vi "Wrapper.vi"(8 "error in":errorcluster, 10 "Actor in":refnum<class "Actor.lvclass">, 11 "Update Heater DC MSG in":refnum<class "Update Heater DC MSG.lvclass">) -> (0 "error out":errorcluster, 3 "Actor out":refnum<class "Actor.lvclass">)   [LabVIEW 2017, in "Controller.lvlib" / "Update Heater DC MSG.lvclass"]
uses:
  Update Heater DC MSG.lvclass
  <vilib>/ActorFramework/Actor/Actor.lvclass
  Update Heater DC MSG.lvclass/Update Heater DC MSG.ctl
  gController.lvclass
  C:/Program Files (x86)/National Instruments/LabVIEW 2017/vi.lib/MSR Consulting, LLC/General Reuse/SuperActor/SuperActor.lvclass
  C:/Program Files (x86)/National Instruments/LabVIEW 2017/vi.lib/ActorFramework/Actor/Actor.lvclass
  <vilib>/MSR Consulting, LLC/General Reuse/SuperActor/SuperActor.lvclass/SuperActor.ctl
  <vilib>/MSR Consulting, LLC/General Reuse/SuperActor/Read CVT Session.vi
  <vilib>/MSR Consulting, LLC/General Reuse/SuperActor/Read Log Session.vi
  Global DO.vi
  <vilib>/Utility/error.llb/Error Cluster From Error Code.vi
  <vilib>/rvi/errors/niLvFpgaAdjustHostInterfaceError.vi
  <vilib>/MSR Consulting, LLC/General Reuse/Session APIs/_Session Fwk/Session - Root.lvclass
  <vilib>/rvi/interface/nirviReadWriteControl/nirviReadWriteControl.xnode
  FPGA Ref.ctl
  FPGA Bitfiles/server.lvbitx
  <vilib>/MSR Consulting, LLC/General Reuse/Session APIs/CVT/CVT.lvclass
  <vilib>/MSR Consulting, LLC/General Reuse/Session APIs/Session Log/System Log.lvclass
  NiFpgaLv.dll
panel:
  out "x-y 3":u32
  out "x-y 2":u32
  out "x+1":i32
  out "x-y":u32
  out "32-bit output":u32
  out "crd":u8
  out "pas2":u8
  out "pas1":u8
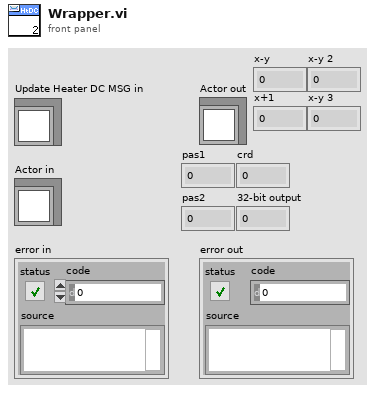
[diagram p1: front panel]
types:
  T1 = typedef "Session - Root.lvclass/Session Handle.ctl" = refnum<data-value>
  T2 = typedef "FPGA Ref.ctl" = refnum<k20>
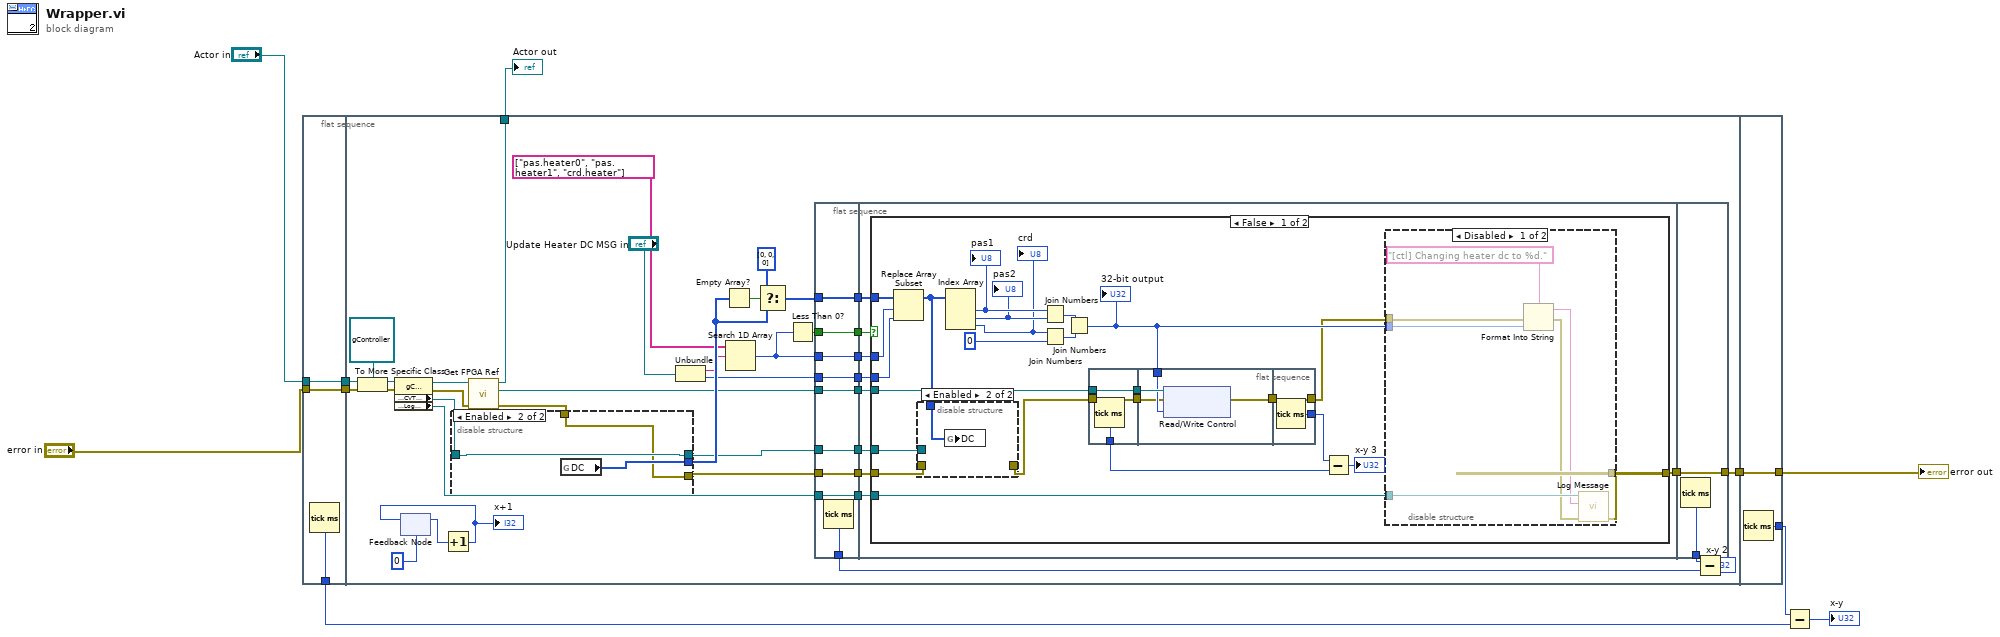
[diagram p0: block diagram]
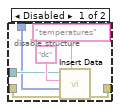
[diagram p3: hidden frame]
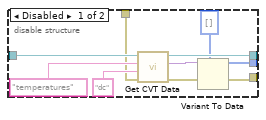
[diagram p5: hidden frame]
diagram:
  n1 = flat-sequence {
    tunnel: "Actor in" -> [w12]
    tunnel: "error in" -> [w13]
    tunnel: [w13] -> w5
    tunnel: [w12] -> w4
    tunnel: [w11] -> w2
    tunnel: [w34] -> w8
    tunnel: [w48] -> w6
    tunnel: w5 -> [w35]
    tunnel: w4 -> [w32]
    tunnel: [w135] -> w10
    tunnel: w6 -> [w135]
    tunnel: [w134] -> w3
    frame #0 {
      n2 = Tick Count (ms)() -> (millisecond timer value=w11:u32)
    }
    frame #1 {
      n3 = To More Specific Class(target class=refnum<class "gController.lvclass"> refnum ("Controller.lvlib:gController"), reference=w32, error in=w35) -> (specific class reference=w38:refnum<class "gController.lvclass">, error out=w39:errorcluster)
      n4 = property class="gController"(reference=w38, error in=w39) -> (reference out=w40:refnum<class "gController.lvclass">, error out=w31:errorcluster, "Accessors:CVT Session"=w41:T1, "Accessors:Log Session"=w49:T1)
      n5 = feedback #1(0) -> (w27:i32)
      n6 = Increment(x=w27) -> (x+1=w26:i32)
      "x+1" <- w26
      n7 = feedback-in #1(w26) -> ()
      n8 = call "Get FPGA Ref.vi"("error in (no error)"=w31, "Actor In"=w40) -> ("error out"=w30:errorcluster, "FPGA Ref"=w36:T2, "Actor Out"=w34:refnum<class "Actor.lvclass">)  [unwired: 7 in]
      n9 = disable-structure shown="Enabled" {
        disable-tunnel: [w130 w133] -> w52
        disable-tunnel: [w129 w132] -> w44
        disable-tunnel: w41 -> [w124 w132]
        disable-tunnel: w30 -> [w123 w131]
        disable-tunnel: [w122 w131] -> w29
        frame Disabled {
          n10 = call <vilib>:"Get CVT Data.vi"("error in"=w123, "Variable"="dc" ("tag"), "Group"="temperatures", "CVT Session In"=w124) -> ("error out"=w122:errorcluster, "Data Out"=w127:variant, "CVT Session Out"=w129:T1)  [unwired: 4 in, 1 out]
          n11 = Variant To Data(type=u8[] [], Variant=w127) -> (data=w130:u8[])  [unwired: 1 in, 1 out]
        }
        frame Enabled {
          n12 = global read "Global DO.vi" "DC"() -> (w133:u8[])
        }
      }
      n13 = Unbundle("Update Heater DC MSG in") -> (w43:string, w45:u8)
      n14 = Empty Array?(array=w52) -> (empty?=w50:bool)
      n15 = Search 1D Array(1D array=string[] ["pas.heater0", "pas.heater1", "crd.heater"], element=w43) -> (index of element=w47:i32)  [unwired: 1 in]
      n16 = Select(t=u8[] [0, 0, 0], s=w50, f=w52) -> (s? t:f=w53:u8[])
      n17 = Less Than 0?(x=w47) -> (x < 0?=w46:bool)
      n18 = flat-sequence {
        tunnel: w29 -> [w55]
        tunnel: w36 -> [w56]
        tunnel: w44 -> [w57]
        tunnel: w45 -> [w58]
        tunnel: w46 -> [w59]
        tunnel: w47 -> [w60]
        tunnel: w49 -> [w61]
        tunnel: w53 -> [w62]
        tunnel: [w62] -> w24
        tunnel: [w61] -> w23
        tunnel: [w60] -> w22
        tunnel: [w59] -> w21
        tunnel: [w58] -> w20
        tunnel: [w57] -> w19
        tunnel: [w56] -> w18
        tunnel: [w55] -> w17
        tunnel: [w54] -> w15
        tunnel: [w69] -> w25
        tunnel: w24 -> [w71]
        tunnel: w23 -> [w70]
        tunnel: w22 -> [w68]
        tunnel: w21 -> [w67]
        tunnel: w20 -> [w66]
        tunnel: w19 -> [w65]
        tunnel: w18 -> [w64]
        tunnel: w17 -> [w63]
        tunnel: [w121] -> w48
        tunnel: w25 -> [w121]
        tunnel: [w120] -> w16
        frame #0 {
          n19 = Tick Count (ms)() -> (millisecond timer value=w54:u32)
        }
        frame #1 {
          n20 = case shown="False" w67 {
            tunnel: w64 -> [w82 _]
            tunnel: w65 -> [w95 _]
            tunnel: w71 -> [w94 _]
            tunnel: w66 -> [w93 _]
            tunnel: w68 -> [w92 _]
            tunnel: [w83 w119] -> w69
            tunnel: w70 -> [w84 _]
            tunnel: w63 -> [w80 w119]
            frame False {
              n21 = Replace Array Subset(array=w94, new element=w93, index=w92) -> (w91:u8[])
              n22 = disable-structure shown="Enabled" {
                disable-tunnel: w95 -> [w115 _]
                disable-tunnel: w91 -> [w114 w118]
                disable-tunnel: w80 -> [w113 _]
                disable-tunnel: [w112 _] -> w79
                frame Disabled {
                  n23 = call <vilib>:"Insert Data.vi"("Group"="temperatures", "error in"=w113, "Data"=w114, "tag"="dc", "CVT Session In"=w115) -> ("error out"=w112:errorcluster)  [unwired: 5 in, 1 out]
                }
                frame Enabled {
                  n24 = global write "Global DO.vi" "DC"(w118) -> ()
                }
              }
              n25 = Index Array(array=w91) -> (element #1=w90:u8, element #2=w89:u8, element #3=w88:u8)  [unwired: 3 in]
              "pas1" <- w90
              "pas2" <- w89
              "crd" <- w88
              n26 = Join Numbers(hi=w90, lo=w89) -> ((hi.lo)=w86:u16)
              n27 = Join Numbers(hi=w88, lo=u8 0) -> ((hi.lo)=w85:u16)
              n28 = Join Numbers(hi=w86, lo=w85) -> ((hi.lo)=w81:u32)
              "32-bit output" <- w81
              n29 = flat-sequence {
                tunnel: w79 -> [w97]
                tunnel: w82 -> [w98]
                tunnel: [w98] -> w76
                tunnel: [w97] -> w75
                tunnel: [w96] -> w73
                tunnel: w81 -> [w101]
                tunnel: [w99] -> w77
                tunnel: w76 -> [w102]
                tunnel: w75 -> [w100]
                tunnel: [w104] -> w78
                tunnel: w77 -> [w104]
                tunnel: [w103] -> w74
                frame #0 {
                  n30 = Tick Count (ms)() -> (millisecond timer value=w96:u32)
                }
                frame #1 {
                  n31 = xnode "Read/Write Control"("FPGA VI Reference In"=w102, "error in"=w100, "HeaterDC"=w101) -> ("error out"=w99:errorcluster)  [unwired: 1 out]
                }
                frame #2 {
                  n32 = Tick Count (ms)() -> (millisecond timer value=w103:u32)
                }
              }
              n33 = Subtract(x=w74, y=w73) -> (x-y=→"x-y 3":u32)
              n34 = disable-structure shown="Disabled" {
                disable-tunnel: w84 -> [w111 _]
                disable-tunnel: [w108 _] -> w83
                disable-tunnel: w81 -> [w107 _]
                disable-tunnel: w78 -> [w106 _]
                frame Disabled {
                  n35 = Format Into String(format string="[ctl] Changing heater dc to %d.", error in=w106, w107) -> (resulting string=w109:string, error out=w105:errorcluster)  [unwired: 1 in]
                  n36 = call <vilib>:"Log Message.vi"("error in"=w105, "MSG In"=w109, "session in"=w111) -> ("error out"=w108:errorcluster)  [unwired: 7 in, 1 out]
                }
                frame Enabled {
                }
              }
            }
            frame True {
            }
          }
        }
        frame #2 {
          n37 = Tick Count (ms)() -> (millisecond timer value=w120:u32)
        }
      }
      n38 = Subtract(x=w16, y=w15) -> (x-y=→"x-y 2":u32)
    }
    frame #2 {
      n39 = Tick Count (ms)() -> (millisecond timer value=w134:u32)
    }
  }
  n40 = Subtract(x=w3, y=w2) -> (x-y=→"x-y":u32)
  "error out" <- w10
  "Actor out" <- w8
